vi "ScoreImage.vi"(0 "Range Params LUTable":cluster{sgl, sgl, sgl, sgl, sgl, sgl} {"?" format="%.2f"; "?" format="%.2f"; "?" format="%.2f"; "?" format="%.2f"; "?" format="%.2f"; "?" format="%.2f"}, 1 "LookUp Table":sgl[][][](array[numeric]) format="%.6f", 2 "fit data":T2, 3 "psa":dbl format="%.2f", 4 "Range Params":T1={"mb max"=-20.0, "mb min"=-70.0, "slope max"=8.0, "slope min"=-8.0, "int max"=5.0, "int min"=-85.0} {"int min" format="%.2f"; "int max" format="%.2f"; "slope min" format="%.2f"; "slope max" format="%.2f"; "mb min" format="%.2f"; "mb max" format="%.2f"}, 5 "window size":i8=3) -> (6 "max score":sgl, 7 "min score":sgl, 8 "score":dbl[][](graph))   [LabVIEW 2022 SP3]
uses:
  <vilib>/Utility/file.llb/Read From Spreadsheet File (DBL).vi
panel:
  in  "lookup path":path
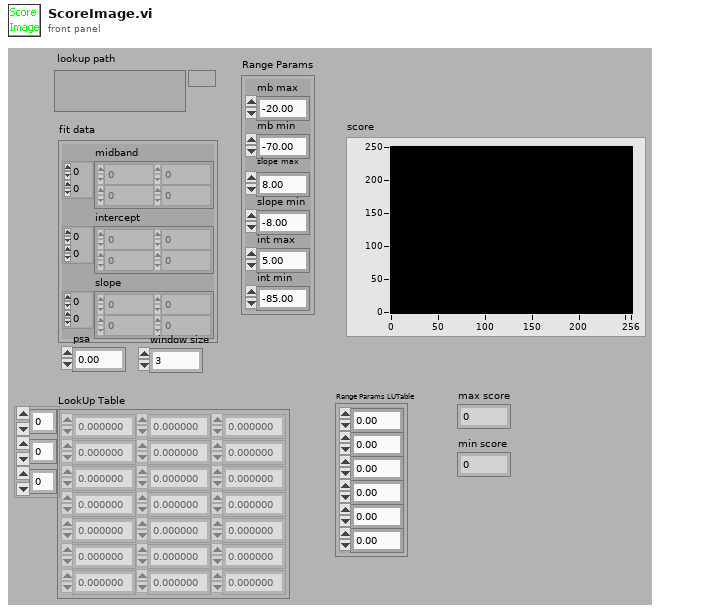
[diagram p1: front panel]
types:
  T1 = cluster{"mb max":dbl, "mb min":dbl, "slope max":dbl, "slope min":dbl, "int max":dbl, "int min":dbl}
  T2 = cluster{"midband":u8[][], "intercept":u8[][], "slope":u8[][]}
  T3 = cluster{"[0]":dbl, "[1]":dbl, "[2]":dbl, "[3]":dbl, "[4]":dbl, "[5]":dbl, "[6]":dbl, "[7]":dbl}
  T4 = cluster{"[5]":dbl, "[4]":dbl, "[1]":dbl, "[0]":dbl, "[3]":dbl, "[2]":dbl}
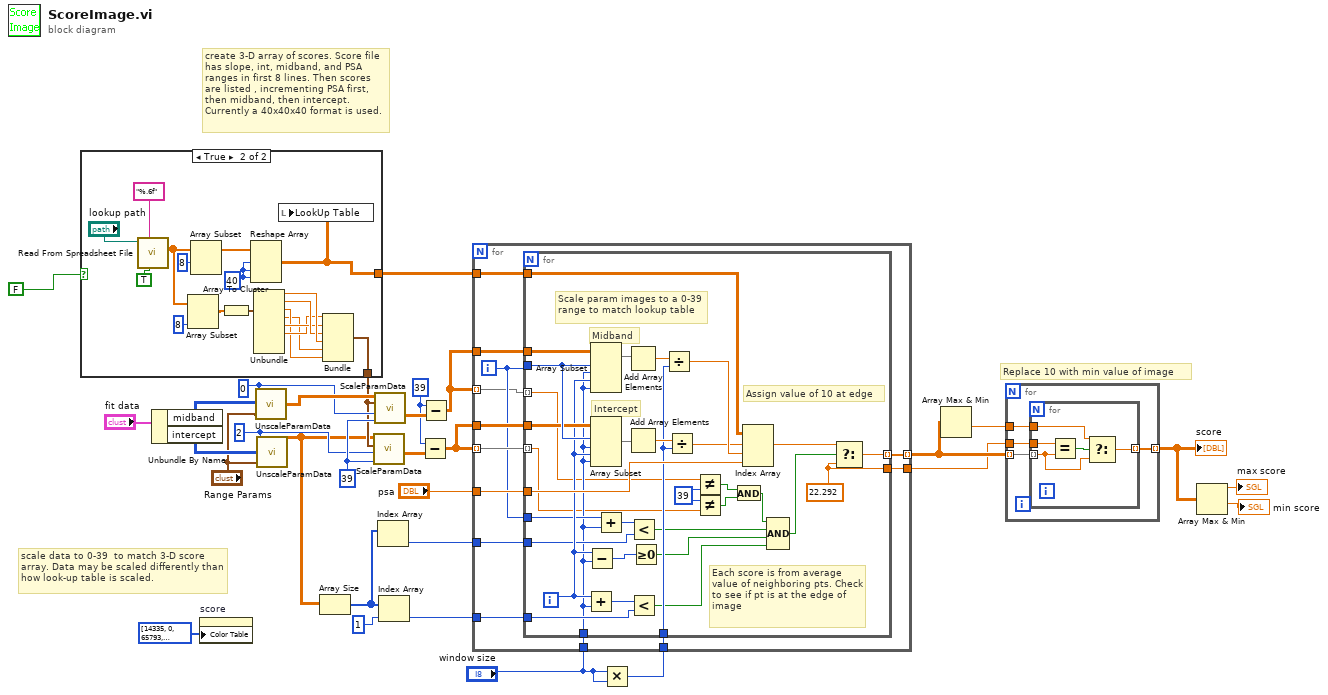
[diagram p0: block diagram]
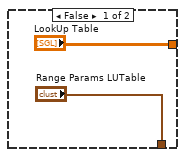
[diagram p2: hidden frame]
diagram:
  w19 = 39
  w25 = 39
  w23 = 2
  w24 = 0
  # "Replace 10 with min value of image"
  # "scale data to 0-39  to match 3-D score array. Data may be scaled differently than how look-up table is scaled."
  # "create 3-D array of scores. Score file has slope, int, midband, and PSA ranges in first 8 lines. Then scores are listed , incrementing PSA first, then midband, then intercept.  Currently a 40x40x40 format is used."
  n1 = case shown="True" FALSE ("Case Constant\n(See Context Help)") {
    tunnel: ["LookUp Table" w34] -> w11
    tunnel: ["Range Params LUTable" w41] -> w22
    frame False {
    }
    frame True {
      w48 = 40
      n2 = call-poly <vilib>:"Read From Spreadsheet File.vi"("transpose (no:F)"=TRUE, "format (%.3f)"="%.6f", "file path (dialog if empty)"="lookup path") -> ("first row"=w47:dbl[])  [unwired: 1 in, 7 out]
      n3 = Array Subset(array=w47, length=8) -> (w45:dbl[])  [unwired: 1 in]
      n4 = Array Subset(array=w47, index=8) -> (w49:dbl[])  [unwired: 1 in]
      n5 = Array To Cluster(array=w45) -> (cluster=w44:T3)
      n6 = Reshape Array(w49, w48, w48, w48) -> (w34:dbl[][][])
      n7 = Unbundle(w44) -> ("[0]"=w43:dbl, "[1]"=w42:dbl, "[2]"=w38:dbl, "[3]"=w37:dbl, "[4]"=w40:dbl, "[5]"=w39:dbl)  [unwired: 2 out]
      n8 = local write "LookUp Table"(w34) -> ()
      n9 = Bundle("[5]"=w39, "[4]"=w40, "[1]"=w42, "[0]"=w43, "[3]"=w37, "[2]"=w38) -> (w41:T4)  [unwired: 1 out]
    }
  }
  n10 = Unbundle By Name("fit data") -> ("midband"=w29:u8[][], "intercept"=w28:u8[][])
  n11 = property on="score" class="IntGraph (strict)"("Color Table"=u32[] [14335, 0, 65793, 131586, 197379, 263172, 328965, 394758, 460551, 526344, 592137, 657930, 723723, 789516, 855309, 921102, 986895, 1052688, 1118481, 1184274, 1250067, 1315860, 1381653, 1447446, 1513239, 1579032, 1644825, 1710618, 1776411, 1842204, 1907997, 1973790, 2039583, 2105376, 2171169, 2236962, 2302755, 2368548, 2434341, 2500134, 2565927, 2631720, 2697513, 2763306, 2829099, 2894892, 2960685, 3026478, 3092271, 3158064, 3223857, 3289650, 3355443, 3421236, 3487029, 3552822, 3618615, 3684408, 3750201, 3815994, 3881787, 3947580, 4013373, 4079166, 4144959, 4210752, 4276545, 4342338, 4408131, 4473924, 4539717, 4605510, 4671303, 4737096, 4802889, 4868682, 4934475, 5000268, 5066061, 5131854, 5197647, 5263440, 5329233, 5395026, 5460819, 5526612, 5592405, 5658198, 5723991, 5789784, 5855577, 5921370, 5987163, 6052956, 6118749, 6184542, 6250335, 6316128, 6381921, 6447714, 6513507, 6579300, 6645093, 6710886, 6776679, 6842472, 6908265, 6974058, 7039851, 7105644, 7171437, 7237230, 7303023, 7368816, 7434609, 7500402, 7566195, 7631988, 7697781, 7763574, 7829367, 7895160, 7960953, 8026746, 8092539, 8158332, 8224125, 8289918, 8355711, 8421504, 8487297, 8553090, 8618883, 8684676, 8750469, 8816262, 8882055, 8947848, 9013641, 9079434, 9145227, 9211020, 9276813, 9342606, 9408399, 9474192, 9539985, 9605778, 9671571, 9737364, 9803157, 9868950, 9934743, 10000536, 10066329, 10132122, 10197915, 10263708, 10329501, 10395294, 10461087, 10526880, 10592673, 10658466, 10724259, 10790052, 10855845, 10921638, 10987431, 11053224, 11119017, 11184810, 11250603, 11316396, 11382189, 11447982, 11513775, 11579568, 11645361, 11711154, 11776947, 11842740, 11908533, 11974326, 12040119, 12105912, 12171705, 12237498, 12303291, 12369084, 12434877, 12500670, 12566463, 12632256, 12698049, 12763842, 12829635, 12895428, 12961221, 13027014, 13092807, 13158600, 13224393, 13290186, 13355979, 13421772, 13487565, 13553358, 13619151, 13684944, 13750737, 13816530, 13882323, 13948116, 14013909, 14079702, 14145495, 14211288, 14277081, 14342874, 14408667, 14474460, 14540253, 14606046, 14671839, 14737632, 14803425, 14869218, 14935011, 15000804, 15066597, 15132390, 15198183, 15263976, 15329769, 15395562, 15461355, 15527148, 15592941, 15658734, 15724527, 15790320, 15856113, 15921906, 15987699, 16053492, 16119285, 16185078, 16250871, 16316664, 16382457, 16448250, 16514043, 16579836, 16758546, 16711731]) -> ()  [unwired: 2 in, 2 out]
  n12 = call "UnscaleParamData.vi"("Range Params"="Range Params", "scaled data"=w29, "Ring"=w24) -> ("UnScaled data"=w26:dbl[][])  [unwired: 1 in]
  n13 = call "UnscaleParamData.vi"("Range Params"="Range Params", "scaled data"=w28, "Ring"=w23) -> ("UnScaled data"=w5:dbl[][])  [unwired: 1 in]
  n14 = Array Size(array=w5) -> (size(s)=w3:i32[])
  n15 = call "ScaleParamData.vi"("max scale value"=w25, "parameter"=w23, "Range Params"=w22, "raw image data in"=w5) -> ("scaled output"=w20:dbl[][])
  n16 = call "ScaleParamData.vi"("max scale value"=w25, "parameter"=w24, "Range Params"=w22, "raw image data in"=w26) -> ("scaled output"=w21:dbl[][])
  n17 = Index Array(array=w3) -> (element=w2:i32)  [unwired: 1 in]
  n18 = Index Array(array=w3, index=1) -> (element=w4:i32)
  n19 = Subtract(x=w19, y=w20) -> (x-y=w6:dbl[][])
  n20 = Subtract(x=w19, y=w21) -> (x-y=w1:dbl[][])
  n21 = Multiply(x="window size", y="window size") -> (x*y=w17:i8)
  n22 = for {
    tunnel: w11 -> [w64]
    tunnel: "psa" -> [w63]
    tunnel: [w62] -> w14 mode=indexing
    tunnel: w1 -> [w61]
    tunnel: w6 -> [w60]
    tunnel: "window size" -> [w59]
    tunnel: w17 -> [w58]
    tunnel: [w57] -> w13
    tunnel: w6 -> [w56] mode=indexing
    tunnel: w4 -> [w55]
    tunnel: w2 -> [w53]
    tunnel: w1 -> [w52] mode=indexing
    i -> [w54]
    n23 = for {
      tunnel: w64 -> [w96]
      tunnel: w63 -> [w97]
      tunnel: [w85] -> w62 mode=indexing
      tunnel: w54 -> [w95]
      tunnel: w61 -> [w94]
      tunnel: w60 -> [w93]
      tunnel: w59 -> [w71]
      tunnel: w58 -> [w81]
      tunnel: [w83] -> w57
      tunnel: w56 -> [w70] mode=indexing
      tunnel: w55 -> [w77]
      tunnel: w54 -> [w74]
      tunnel: w53 -> [w73]
      tunnel: w52 -> [w69] mode=indexing
      i -> [w86]
      w68 = 39
      w83 = 22.292
      # "Assign value of 10 at edge"
      # "Scale param images to a 0-39 range to match lookup table"
      # "Each score is from average value of neighboring pts. Check to see if pt is at the edge of image"
      # "Intercept"
      # "Midband"
      n24 = Add(x=w86, y=w71) -> (x+y=w78:i32)
      n25 = Subtract(x=w86, y=w71) -> (x-y=w80:i32)
      n26 = Array Subset(array=w94, index (row)=w95, length (row)=w71, index (col)=w86, length (col)=w71) -> (w92:dbl[][])
      n27 = Array Subset(array=w93, index (row)=w95, length (row)=w71, index (col)=w86, length (col)=w71) -> (w91:dbl[][])
      n28 = Add(x=w74, y=w71) -> (x+y=w75:i32)
      n29 = Add Array Elements(numeric array=w92) -> (sum=w89:dbl)
      n30 = Add Array Elements(numeric array=w91) -> (sum=w90:dbl)
      n31 = Less?(x=w75, y=w73) -> (x < y?=w72:bool)
      n32 = Less?(x=w78, y=w77) -> (x < y?=w76:bool)
      n33 = Greater Or Equal To 0?(x=w80) -> (x >= 0?=w79:bool)
      n34 = Divide(x=w89, y=w81) -> (x/y=w88:dbl)
      n35 = Divide(x=w90, y=w81) -> (x/y=w87:dbl)
      n36 = Not Equal?(x=w69, y=w68) -> (x != y?=w67:bool)
      n37 = Not Equal?(x=w68, y=w70) -> (x != y?=w66:bool)
      n38 = And(x=w67, y=w66) -> (x .and. y?=w65:bool)
      n39 = Index Array(array=w96, index (dim 0)=w87, index (dim 1)=w88, index (dim 2)=w97) -> (element=w84:dbl)
      n40 = Compound Arithmetic op=AND(w65, w72, w79, w76) -> (w82:bool)
      n41 = Select(t=w84, s=w82, f=w83) -> (s? t:f=w85:dbl)
    }
  }
  n42 = Array Max & Min(array=w14) -> (min value=w15:dbl)  [unwired: 3 out]
  n43 = for {
    tunnel: [w101] -> w10 mode=indexing
    tunnel: w14 -> [w100] mode=indexing
    tunnel: w13 -> [w99]
    tunnel: w15 -> [w98]
    n44 = for {
      tunnel: [w105] -> w101 mode=indexing
      tunnel: w100 -> [w102] mode=indexing
      tunnel: w99 -> [w104]
      tunnel: w98 -> [w103]
      n45 = Equal?(x=w104, y=w102) -> (x = y?=w106:bool)
      n46 = Select(t=w103, s=w106, f=w102) -> (s? t:f=w105:dbl)
    }
  }
  "score" <- w10
  n47 = Array Max & Min(array=w10) -> (max value=→"max score":dbl, min value=→"min score":dbl)  [unwired: 2 out]
